vi "Event Notification.Set Logging Level.vi"(10 "Log Level":T1, 11 "Event Notification in":refnum<class "Event Notification.lvclass">) -> (3 "Event Notification out":refnum<class "Event Notification.lvclass">)   [LabVIEW 2024, in "EQMF.lvlib" / "Event Log.lvlib" / "Event Notification.lvclass"]
uses:
  Event Notification.lvclass
  Event Log.Log Level.ctl
  Event Notification.lvclass/Event Notification.ctl
  Event Log.lvlib
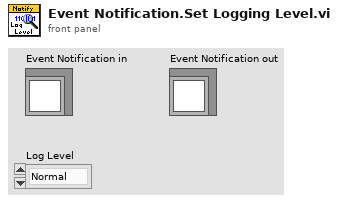
[diagram p1: front panel]
types:
  T1 = typedef "EQMF.lvlib/Event Log.lvlib/Event Log.Log Level.ctl" = enum16{"Normal", "Verbose", "Debug0", "Debug1", "Debug2"}
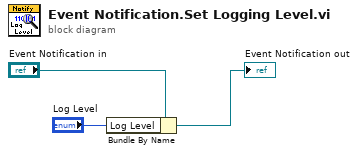
[diagram p0: block diagram]
diagram:
  n1 = Bundle By Name(cluster="Event Notification in", "Log Level"="Log Level") -> (→"Event Notification out":refnum<class "Event Notification.lvclass">)
